vi "SaveFinger.vi"(8 "error in (no error)":errorcluster, 11 "Finger Refnum":refnum<k24>) -> (0 "error out":errorcluster, 3 "Finger":T1)   [LabVIEW 2017, in "LeapMotion.lvlib"]
uses:
  LeapMotion.lvlib
  TypeDefs/LEAPfinger.ctl
  TypeDefs/LEAPvector.ctl
  TypeDefs/LEAPbone.ctl
  C:/Users/snordinh/Desktop/LEAP/LEAP-sign-language-test/LeapMotion/Dynamic Libraries/LeapCSharp.NET4.5.dll
  Dynamic Libraries/LeapCSharp.NET4.5.dll
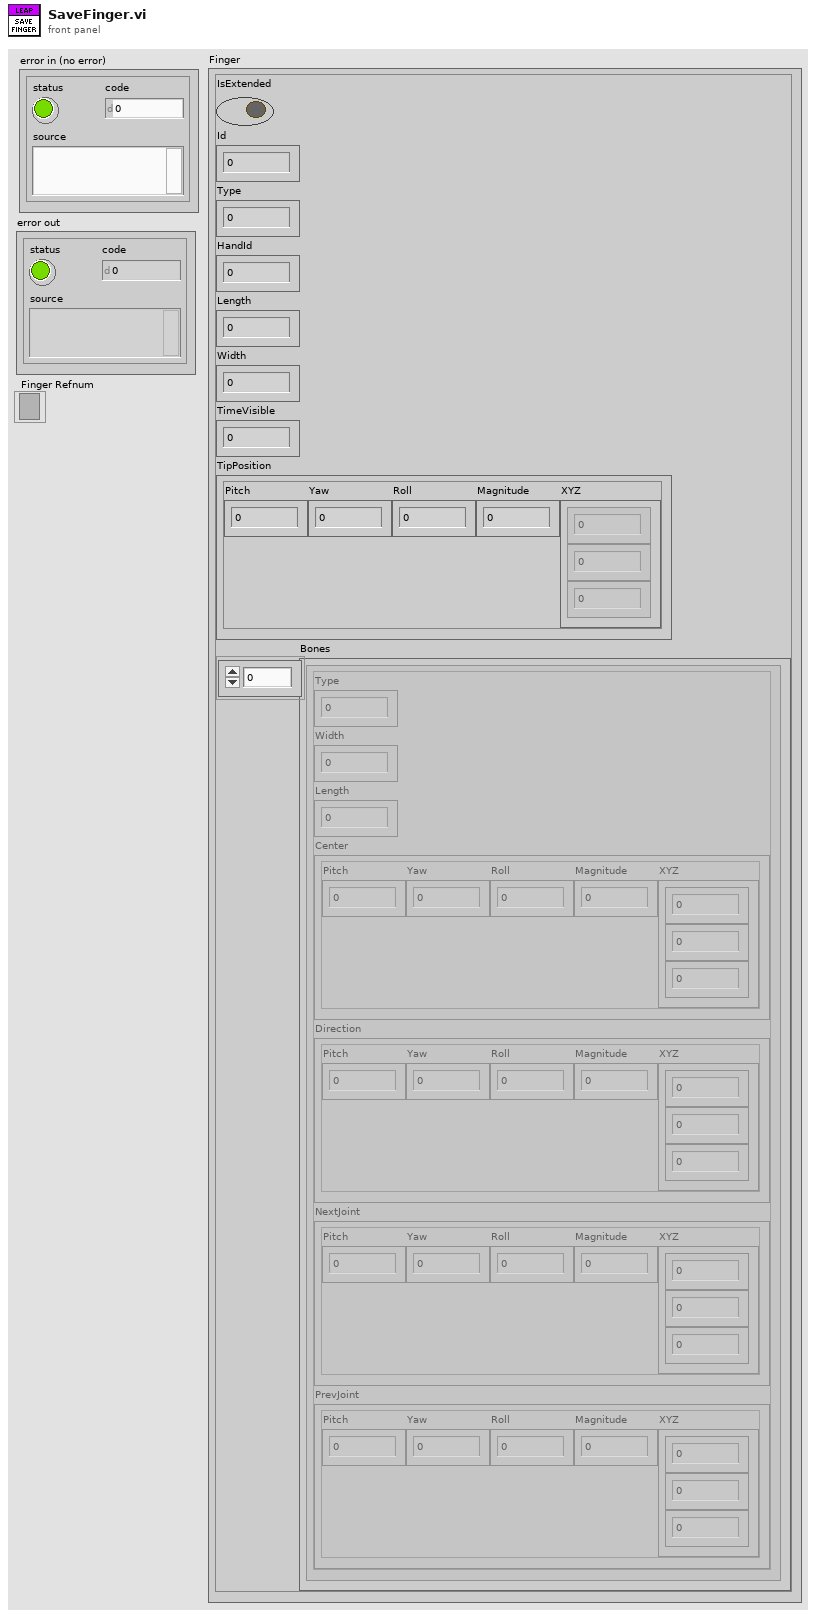
[diagram p1: front panel]
types:
  T1 = typedef "LeapMotion.lvlib/LEAPfinger.ctl" = cluster{"IsExtended":bool, "Id":i32, "Type":i32, "HandId":i32, "Length":sgl, "Width":sgl, "TimeVisible":sgl, "TipPosition":T2, "Bones":T3[]}
  T2 = typedef "LeapMotion.lvlib/LEAPvector.ctl" = cluster{"Pitch":sgl, "Yaw":sgl, "Roll":sgl, "Magnitude":sgl, "XYZ":sgl[]}
  T3 = typedef "LeapMotion.lvlib/LEAPbone.ctl" = cluster{"Type":i32, "Width":sgl, "Length":sgl, "Center":T2, "Direction":T2, "NextJoint":T2, "PrevJoint":T2}
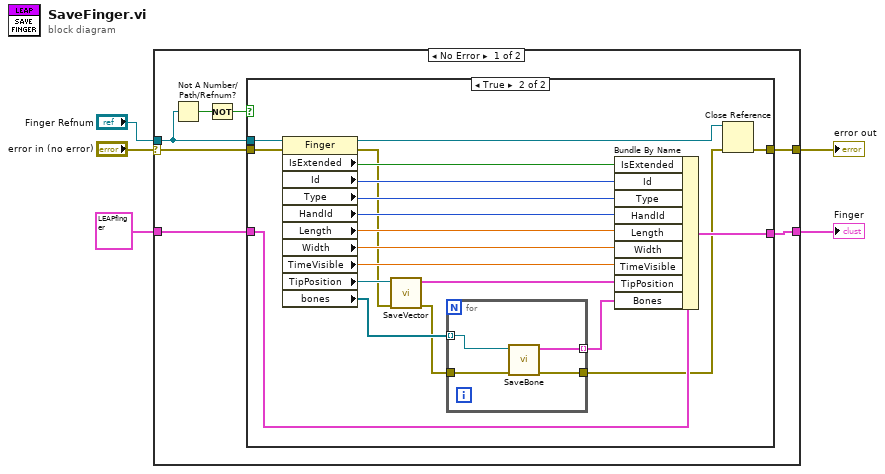
[diagram p0: block diagram]
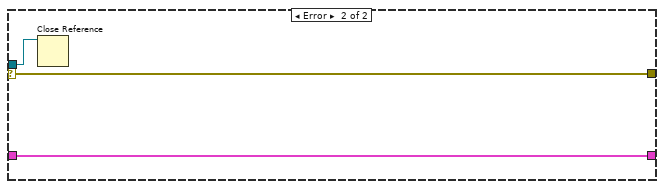
[diagram p3: hidden frame]
diagram:
  n1 = case shown="No Error" "error in (no error)" {
    selector: "error in (no error)" -> [w6 w39]
    tunnel: [w12 w39] -> w1
    tunnel: "Finger Refnum" -> [w7 w41]
    tunnel: [w11 w40] -> w3
    tunnel: T1 {"IsExtended"=FALSE, "Id"=0, "Type"=0, "HandId"=0, "Length"=0.0, "Width"=0.0, "TimeVisible"=0.0, "TipPosition"={"Pitch"=0.0, "Yaw"=0.0, "Roll"=0.0, "Magnitude"=0.0, "XYZ"=[]}, "Bones"=[]} ("Finger") -> [w10 w40]
    frame No Error {
      n2 = Not A Number/Path/Refnum?(number/path/refnum=w7) -> (NaN/Path/Refnum?=w9:bool)
      n3 = Not(x=w9) -> (.not. x?=w8:bool)
      n4 = case shown="True" w8 {
        tunnel: [w14 w15] -> w12
        tunnel: w6 -> [w14 w34]
        tunnel: w7 -> [_ w33]
        tunnel: [w13 w19] -> w11
        tunnel: w10 -> [w13 w18]
        frame False {
        }
        frame True {
          n5 = property class="Finger"(reference=w33, error in=w34) -> (reference out=w17:refnum<k24>, error out=w22:errorcluster, "IsExtended"=w31:bool, "Id"=w30:i32, "Type"=w29:i32, "HandId"=w28:i32, "Length"=w27:sgl, "Width"=w26:sgl, "TimeVisible"=w25:sgl, "TipPosition"=w24:refnum<k24>, "bones"=w32:refnum<k24>[])
          n6 = call "SaveVector.vi"("error in (no error)"=w22, "Vector Refnum"=w24) -> ("error out"=w21:errorcluster, "LEAPvector"=w23:T2)  [unwired: 8 in]
          n7 = for {
            tunnel: w32 -> [w35] mode=indexing
            tunnel: [w36] -> w20 mode=indexing
            tunnel: w21 -> [w37]
            tunnel: [w38] -> w16
            n8 = call "SaveBone.vi"("error in (no error)"=w37, "Bone Refnum"=w35) -> ("error out"=w38:errorcluster, "Bone"=w36:T3)  [unwired: 8 in]
          }
          n9 = Bundle By Name(cluster=w18, "IsExtended"=w31, "Id"=w30, "Type"=w29, "HandId"=w28, "Length"=w27, "Width"=w26, "TimeVisible"=w25, "TipPosition"=w23, "Bones"=w20) -> (w19:T1)
          n10 = Close Reference(reference=w17, error in (no error)=w16) -> (error out=w15:errorcluster)
        }
      }
    }
    frame Error {
      n11 = Close Reference(reference=w41) -> ()  [unwired: 1 in, 1 out]
    }
  }
  "Finger" <- w3
  "error out" <- w1
